vi "PID setpoint no reset.vi"(4 "State":i16, 5 "Time":dbl format="%.2f", 6 "Sensor Values":dbl[](array[numeric]), 7 "Set Points":dbl[](array[numeric])) -> (0 "required data":T1={"Set Point names"=["target value", "P Kc", "I Ti (min)", "D Td (min)", "Measured process value"], "required number of setpoints"=5, "required number of sensors"=0, "Sensor names"=[]}, 3 "output value":dbl)   [LabVIEW 2019]
uses:
  <vilib>/addons/control/pid/pid.llb/PID (DBL).vi
  <vilib>/addons/control/pid/NI_PID_pid.lvlib
panel:
  # "Enter the correct information for this control code in the required data structure below. Then make the current value default by right clicking on the border of the data structure."
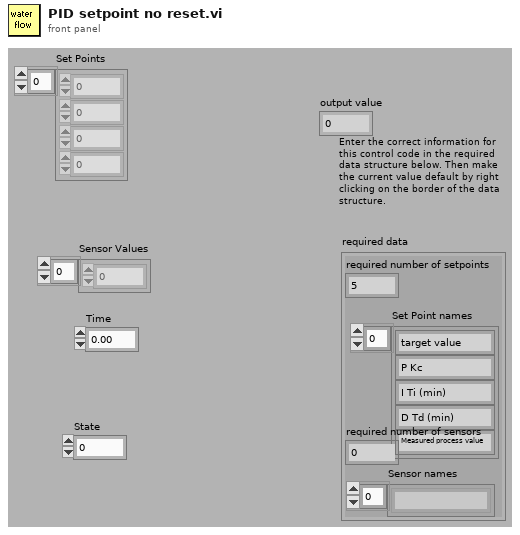
[diagram p1: front panel]
types:
  T1 = cluster{"Set Point names":string[], "required number of setpoints":u8, "required number of sensors":u8, "Sensor names":string[]}
  T2 = cluster{"Set Points[0]":dbl, "Set Points[1]":dbl, "Set Points[2]":dbl, "Set Points[3]":dbl, "Set Points[4]":dbl}
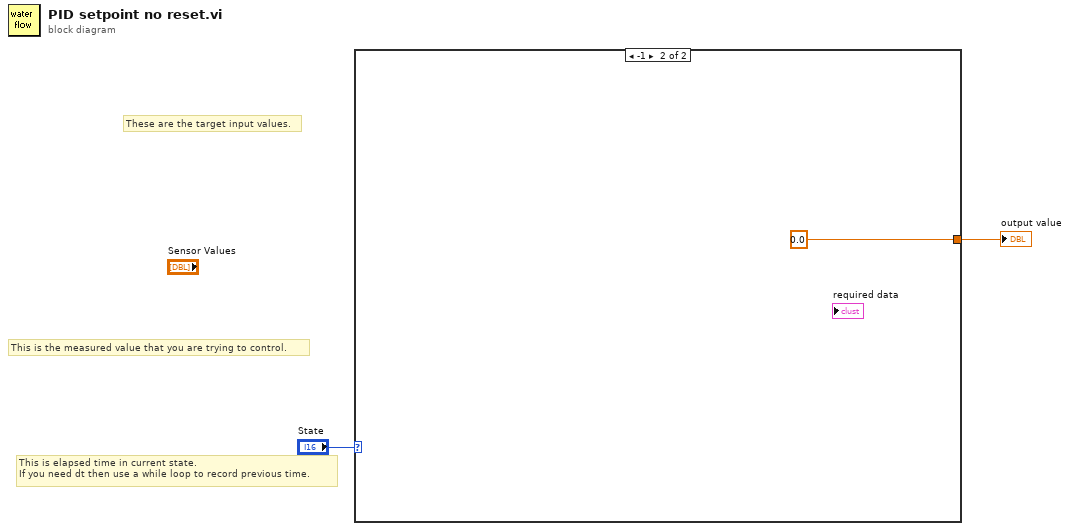
[diagram p0: block diagram]
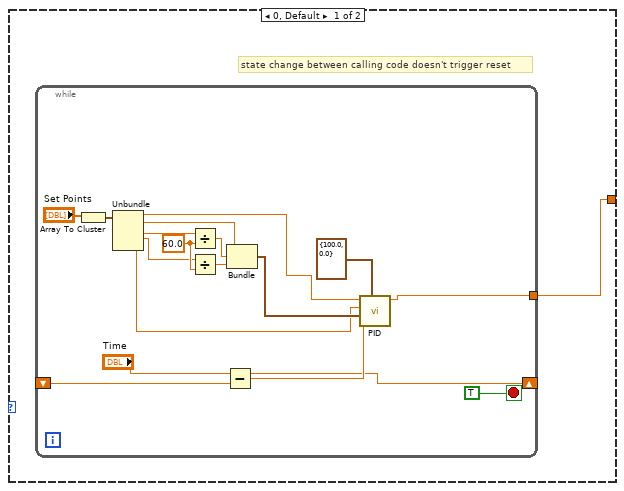
[diagram p2: hidden frame]
diagram:
  # "These are the target input values."
  # "This is the measured value that you are trying to control."
  # "This is elapsed time in current state.\nIf you need dt then use a while loop to record previous time."
  n1 = case shown="-1" "State" {
    tunnel: [w3 0.0 ("fraction on")] -> w2
    frame 0, Default {
      # "state change between calling code doesn't trigger reset"
      n2 = while {
        shift-right: ["Time"] -> _
        shift-left: _ -> [w20]
        tunnel: [w9] -> w3
        stop <- TRUE stop-if-true
        w8 = 60.0 ("y")
        n3 = Array To Cluster(array="Set Points") -> (cluster=w15:T2)
        n4 = Unbundle(w15) -> ("Set Points[0]"=w11:dbl, "Set Points[1]"=w14:dbl, "Set Points[2]"=w5:dbl, "Set Points[3]"=w7:dbl, "Set Points[4]"=w10:dbl)
        n5 = Divide(x=w5, y=w8) -> (x/y=w4:dbl)
        n6 = Divide(x=w7, y=w8) -> (x/y=w6:dbl)
        n7 = Subtract(x="Time", y=w20) -> (x-y=w19:dbl)
        n8 = Bundle("Set Points[1]"=w14, w4, w6) -> (w13:cluster{"Set Points[1]":dbl, dbl, dbl})  [unwired: 1 in]
        n9 = call-poly <vilib>:"PID.vi"("output range"=cluster{"output high":dbl, "output low":dbl} {"output high"=100.0, "output low"=0.0}, "dt (s)"=w19, "PID gains"=w13, "process variable"=w10, "setpoint"=w11) -> ("output"=w9:dbl)  [unwired: 5 in, 1 out]
      }
    }
    frame -1 {
    }
  }
  "output value" <- w2
